vi "Enqueue Multiple States.vi"(0 "State(s) at Front":string, 5 "queue in":refnum<queue>, 7 "State(s) at Back":string) -> (6 "queue out":refnum<queue>)   [LabVIEW 2020, in "MacroAssert.lvlib" / "FaKI State Machine.lvlib"]
doc: "Adds states to the front and/or back of the queue. Use \"Enqueue Element.vi\" and \"Enqueue Element at Opposite End.vi\" instead of this if there is data to be bundled with the state.\n\nCurrently, if this is used to enqueue multiple states at the opposite end from the Producer Loop, unexpected behavior can result."
uses:
  FaKI State Machine.lvlib
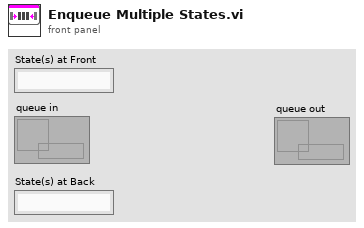
[diagram p1: front panel]
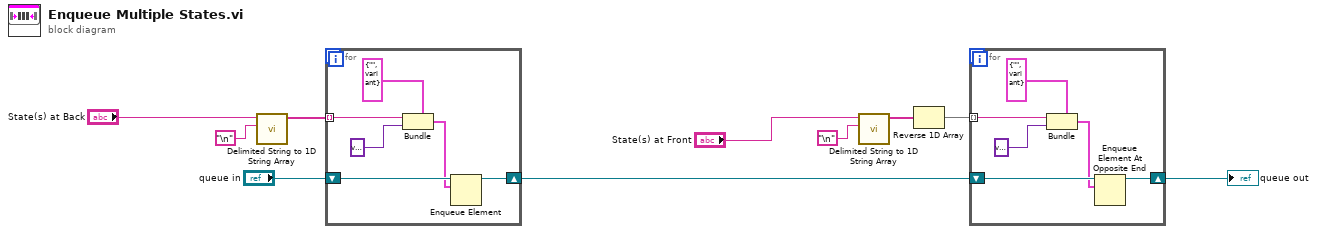
[diagram p0: block diagram]
diagram:
  n1 = call <vilib>:"Delimited String to 1D String Array.vi"("delimiter"="\n", "delimited string"="State(s) at Back") -> ("string array"=w6:string[])  [unwired: 9 in]
  n2 = for {
    tunnel: w6 -> [w15] mode=indexing
    shift-right: [w12] -> w9
    shift-left: "queue in" -> [w13]
    n3 = Bundle(cluster=cluster{string, variant} {"", variant} ("element"), w15, variant) -> (w11:cluster{string, variant})
    n4 = Enqueue Element(queue=w13, element=w11) -> (queue out=w12:refnum<queue>)  [unwired: 2 in, 2 out]
  }
  n5 = call <vilib>:"Delimited String to 1D String Array.vi"("delimiter"="\n", "delimited string"="State(s) at Front") -> ("string array"=w2:string[])  [unwired: 9 in]
  n6 = Reverse 1D Array(array=w2) -> (reversed array=w1:string[])
  n7 = for {
    tunnel: w1 -> [w21] mode=indexing
    shift-right: [w18] -> w8
    shift-left: w9 -> [w19]
    n8 = Bundle(cluster=cluster{string, variant} {"", variant} ("element"), w21, variant) -> (w17:cluster{string, variant})
    n9 = Enqueue Element At Opposite End(queue=w19, element=w17) -> (queue out=w18:refnum<queue>)  [unwired: 2 in, 2 out]
  }
  "queue out" <- w8
